vi "Configure Reading Buffer Mode.vi"(0 "VISA resource name":refnum<visa-resource-name>, 1 "Data Fill Count (0)":i32, 2 "Data Fill Mode (0: Fill Once)":i32(ring) items=["Fill Once", "Fill Window"], 5 "Source Measure Unit Channel (0: Channel A)":i32(ring) items=["Channel A", "Channel B"], 7 "Reading Buffer (smua.nvbuffer1)":string="smua.nvbuffer1", 9 "Enable Data Append (F: Disable)":bool, 11 "error in (no error)":errorcluster, 12 "Enable Data Cache (T: Enable)":bool=TRUE) -> (4 "VISA resource name out":refnum<visa-resource-name>, 15 "error out":errorcluster)   [LabVIEW 2020, in "Keithley 2600 Series.lvlib"]
doc: "Configures the basic settings of the reading buffer.\n\n<b>Note:</b>\nThis VI also clears the buffer data and cache data."
uses:
  <instrlib>/Keithley 2600 Series/Keithley 2600 Series.lvlib
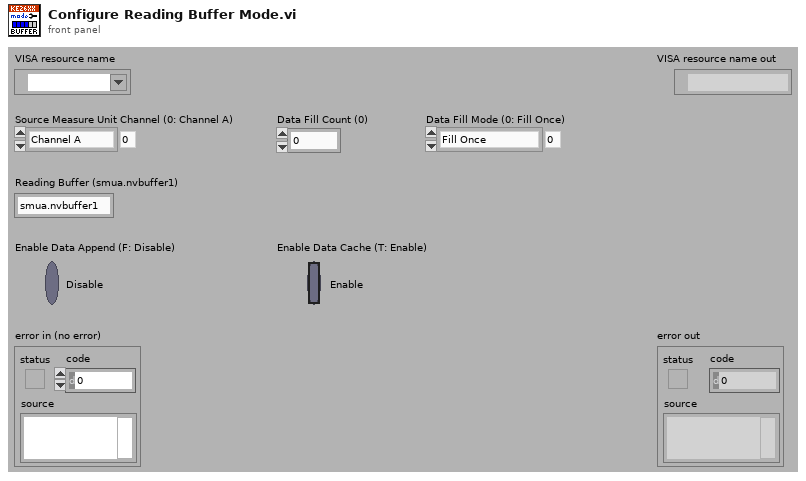
[diagram p1: front panel]
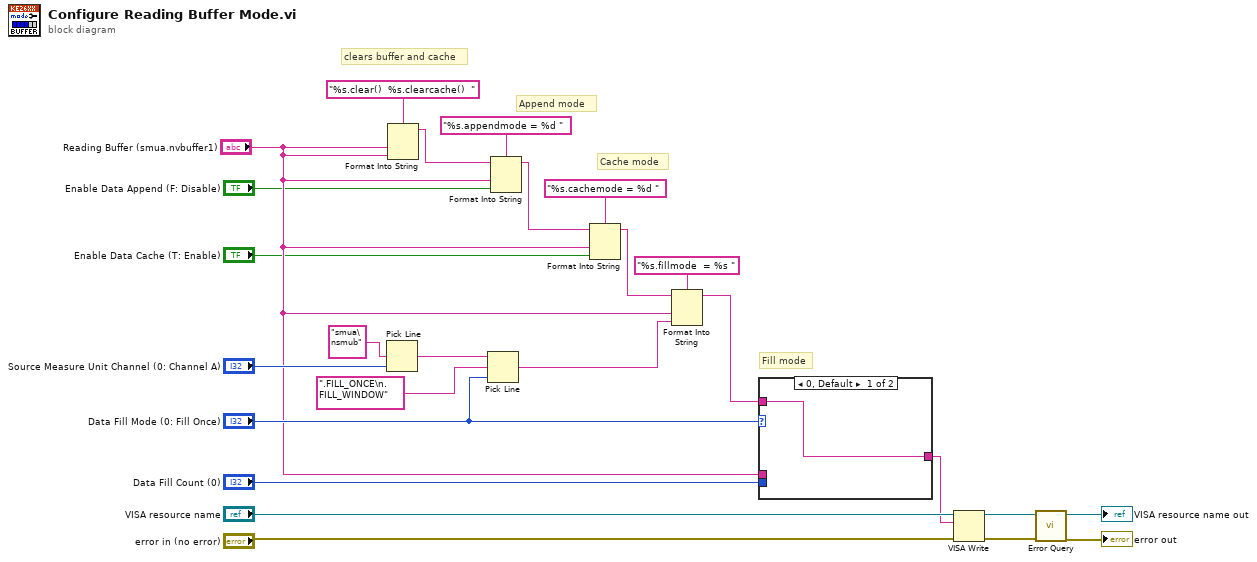
[diagram p0: block diagram]
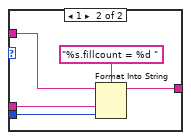
[diagram p2: hidden frame]
diagram:
  # "clears buffer and cache"
  # "Fill mode"
  # "Cache mode"
  # "Append mode"
  n1 = Pick Line(multi-line string="smua\nsmub", line index="Source Measure Unit Channel (0: Channel A)") -> (output string=w12:string)  [unwired: 1 in]
  n2 = Format Into String(format string="%s.clear()  %s.clearcache()  ", "Reading Buffer (smua.nvbuffer1)", "Reading Buffer (smua.nvbuffer1)") -> (resulting string=w4:string)  [unwired: 2 in, 1 out]
  n3 = Pick Line(string ("")=w12, multi-line string=".FILL_ONCE\n.FILL_WINDOW", line index="Data Fill Mode (0: Fill Once)") -> (output string=w11:string)
  n4 = Format Into String(format string="%s.appendmode = %d ", initial string=w4, "Reading Buffer (smua.nvbuffer1)", "Enable Data Append (F: Disable)") -> (resulting string=w16:string)  [unwired: 1 in, 1 out]
  n5 = Format Into String(format string="%s.cachemode = %d ", initial string=w16, "Reading Buffer (smua.nvbuffer1)", "Enable Data Cache (T: Enable)") -> (resulting string=w9:string)  [unwired: 1 in, 1 out]
  n6 = Format Into String(format string="%s.fillmode  = %s ", initial string=w9, "Reading Buffer (smua.nvbuffer1)", w11) -> (resulting string=w7:string)  [unwired: 1 in, 1 out]
  n7 = case shown="0, Default" "Data Fill Mode (0: Fill Once)" {
    tunnel: "Data Fill Count (0)" -> [_ w30]
    tunnel: "Reading Buffer (smua.nvbuffer1)" -> [_ w29]
    tunnel: w7 -> [w26 w28]
    tunnel: [w26 w27] -> w6
    frame 0, Default {
    }
    frame 1 {
      n8 = Format Into String(format string="%s.fillcount = %d ", initial string=w28, w29, w30) -> (resulting string=w27:string)  [unwired: 1 in, 1 out]
    }
  }
  n9 = VISA Write(VISA resource name="VISA resource name", write buffer=w6, error in (no error)="error in (no error)") -> (VISA resource name out=w20:refnum<visa-resource-name>, error out=w19:errorcluster)  [unwired: 1 out]
  n10 = call <instrlib>:"Error Query.vi"("error in (no error)"=w19, "VISA resource name"=w20) -> ("error out"=→"error out":errorcluster, "VISA resource name out"=→"VISA resource name out":refnum<visa-resource-name>)  [unwired: 6 in, 2 out]
